vi "Nested Aliases Wrapper.vi"(11 "Dev Actor in":refnum<class "Dev Actor.lvclass">) -> (0 "error out":errorcluster, 2 "Nested Aliases":string[](array[string]))   [LabVIEW 2021, in "Dev Actor.lvlib" / "Dev Actor.lvclass"]
uses:
  Dev Actor.lvclass
  Dev Actor.lvclass/Dev Actor.ctl
  LVCAM/LVCAM/Actor/Actor.lvclass
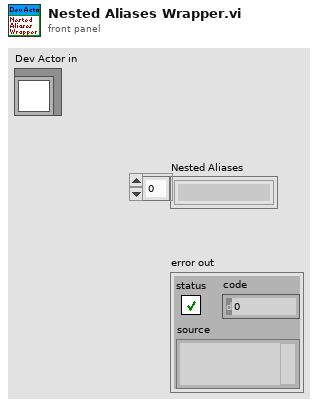
[diagram p1: front panel]
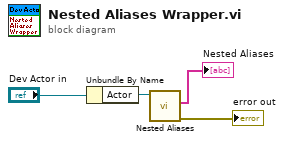
[diagram p0: block diagram]
diagram:
  n1 = Unbundle By Name("Dev Actor in") -> ("Actor"=w3:refnum<class "Actor.lvclass">)
  n2 = call-dynamic "Nested Aliases.vi"("Actor in"=w3) -> ("error out"=→"error out":errorcluster, "Nested Aliases"=→"Nested Aliases":string[])  [unwired: 9 in]
